vi "Unflatten.vi"(8 "error in (no error)":errorcluster, 11 "Analog Out Scan in":refnum<class "Analog Out Scan.lvclass">) -> (0 "error out":errorcluster, 3 "Analog Out Scan out":refnum<class "Analog Out Scan.lvclass">)   [LabVIEW 2009, in "Analog Out Scan.lvclass"]
uses:
  Analog Out Scan.lvclass
  Scanner/Scanner.lvclass
  Global/File Locations.vi
  Analog Out Scan.lvclass/Analog Out Scan.ctl
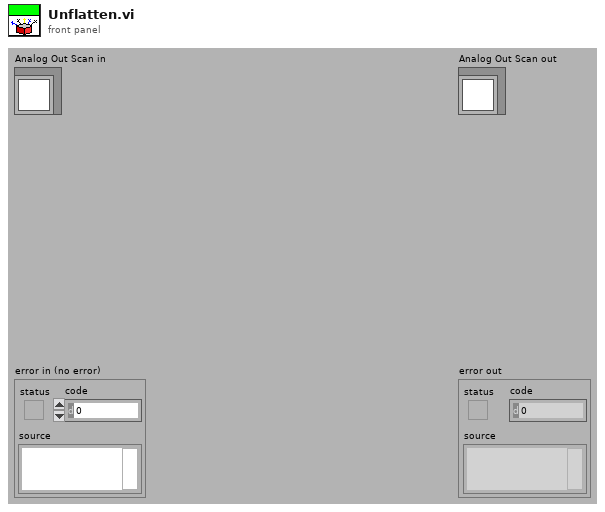
[diagram p1: front panel]
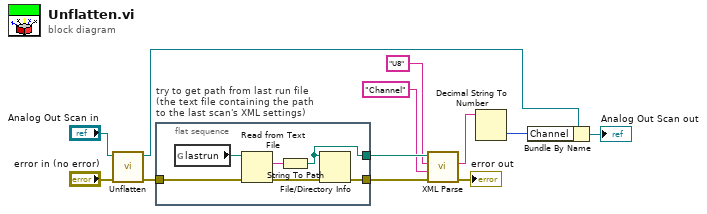
[diagram p0: block diagram]
diagram:
  n1 = call-parent "Unflatten.vi"("error in (no error)"="error in (no error)", "Scanner in"="Analog Out Scan in") -> ("error out"=w9:errorcluster, "Scanner out"=w12:refnum<class "Analog Out Scan.lvclass">)  [unwired: 8 in]
  n2 = flat-sequence "try to get path from last run file\n(the text file containing the path\nto the last scan's XML settings)" {
    tunnel: [w18] -> w7
    tunnel: [w14] -> w4
    tunnel: w9 -> [w13]
    frame #0 {
      n3 = global read "File Locations.vi" "lastrun"() -> (w16:path)
      n4 = Read from Text File(file (use dialog)=w16, error in=w13) -> (text=w17:string, error out=w15:errorcluster)  [unwired: 4 out]
      n5 = String To Path(string=w17) -> (path=w18:path)
      n6 = File/Directory Info(path=w18, error in=w15) -> (error out=w14:errorcluster)  [unwired: 6 out]
    }
  }
  n7 = call "XML Parse.vi"("error in (no error)"=w4, "Name String"="Channel", "Type String"="U8", "Path"=w7) -> ("error out"=→"error out":errorcluster, "String Out"=w2:string)  [unwired: 6 in]
  n8 = Decimal String To Number(string=w2) -> (number=w1:i32)  [unwired: 2 in, 1 out]
  n9 = Bundle By Name(cluster=w12, "Channel"=w1) -> (→"Analog Out Scan out":refnum<class "Analog Out Scan.lvclass">)
